vi "ComponentSimulatorsLauncher.vi"() -> ()   [LabVIEW 2018]
doc: "This launches both Component Simulator A and B."
uses:
  src/TcpServer/configServerTypeDef.ctl
  src/TcpServerTel/typedef/enqueueOptionsTypeDef.ctl
  src/FactoryTcpServer/FactoryTcpServer.lvclass
  src/TcpServerTel/TcpServerTel.lvclass
  src/TcpServer/TcpServer.lvclass
panel:
  out "error out B":errorcluster
  out "error out A":errorcluster
  in  "error in (no error)":errorcluster
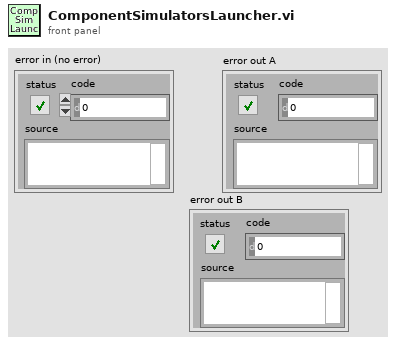
[diagram p1: front panel]
types:
  T1 = typedef "TcpServer.lvclass/configServerTypeDef.ctl" = cluster{"cmdServerPort":u16, "telServerPort":u16, "timeoutServerInMs":i32, "serverBytesToRead":i32, "maxSizeQueueTcpClientFromDds":i32, "EnqueueOptions":T2, "timeoutQueueTcpClientFromDds (ms)":i32, "maxSizeQueueTcpClient":i32, "timeoutInMs":i32}
  T2 = typedef "TcpServerTel.lvclass/enqueueOptionsTypeDef.ctl" = enum16{"lossy enqueue", "normal enqueue"}
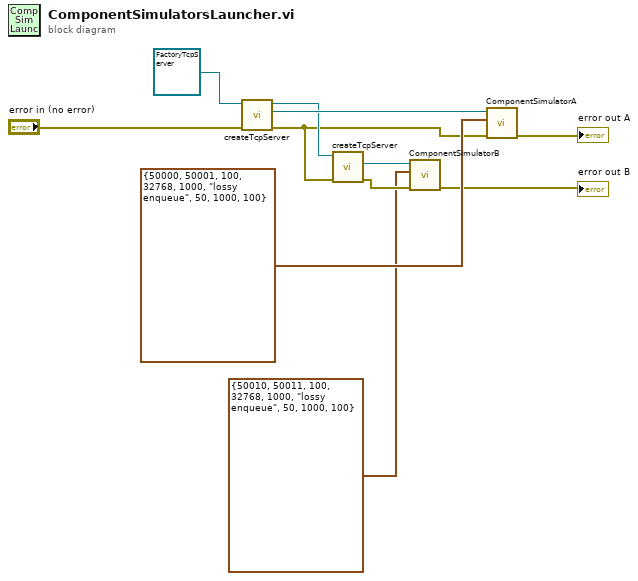
[diagram p0: block diagram]
diagram:
  n1 = call "createTcpServer.vi"("error in (no error)"="error in (no error)", "FactoryTcpServer in"=refnum<class "FactoryTcpServer.lvclass"> refnum ("FactoryTcpServer.lvclass")) -> ("error out"=w4:errorcluster, "TcpServer out"=w9:refnum<class "TcpServer.lvclass">, "FactoryTcpServer out"=w7:refnum<class "FactoryTcpServer.lvclass">)  [unwired: 7 in]
  n2 = call "createTcpServer.vi"("error in (no error)"=w4, "FactoryTcpServer in"=w7) -> ("error out"=w5:errorcluster, "TcpServer out"=w6:refnum<class "TcpServer.lvclass">)  [unwired: 7 in, 1 out]
  n3 = call "ComponentSimulatorB.vi"("error in"=w5, "ServerConfiguration"=T1 {"cmdServerPort"=50010, "telServerPort"=50011, "timeoutServerInMs"=100, "serverBytesToRead"=32768, "maxSizeQueueTcpClientFromDds"=1000, "EnqueueOptions"=enum."lossy enqueue", "timeoutQueueTcpClientFromDds (ms)"=50, "maxSizeQueueTcpClient"=1000, "timeoutInMs"=100}, "tcpServer in"=w6) -> ("error out"=→"error out B":errorcluster)  [unwired: 8 in]
  n4 = call "ComponentSimulatorA.vi"("error in"=w4, "ServerConfiguration"=T1 {"cmdServerPort"=50000, "telServerPort"=50001, "timeoutServerInMs"=100, "serverBytesToRead"=32768, "maxSizeQueueTcpClientFromDds"=1000, "EnqueueOptions"=enum."lossy enqueue", "timeoutQueueTcpClientFromDds (ms)"=50, "maxSizeQueueTcpClient"=1000, "timeoutInMs"=100}, "tcpServer in"=w9) -> ("error out"=→"error out A":errorcluster)  [unwired: 8 in]
